vi "Layout Badges.vi"(8 "error in (no error)":errorcluster, 11 "Node in":refnum<class "FSM.Node.lvclass">) -> (0 "error out":errorcluster, 3 "Node out":refnum<class "FSM.Node.lvclass">)   [LabVIEW 2015, in "FSM.Node.lvclass"]
uses:
  FSM.Node.lvclass
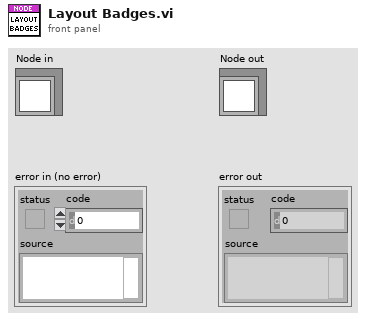
[diagram p1: front panel]
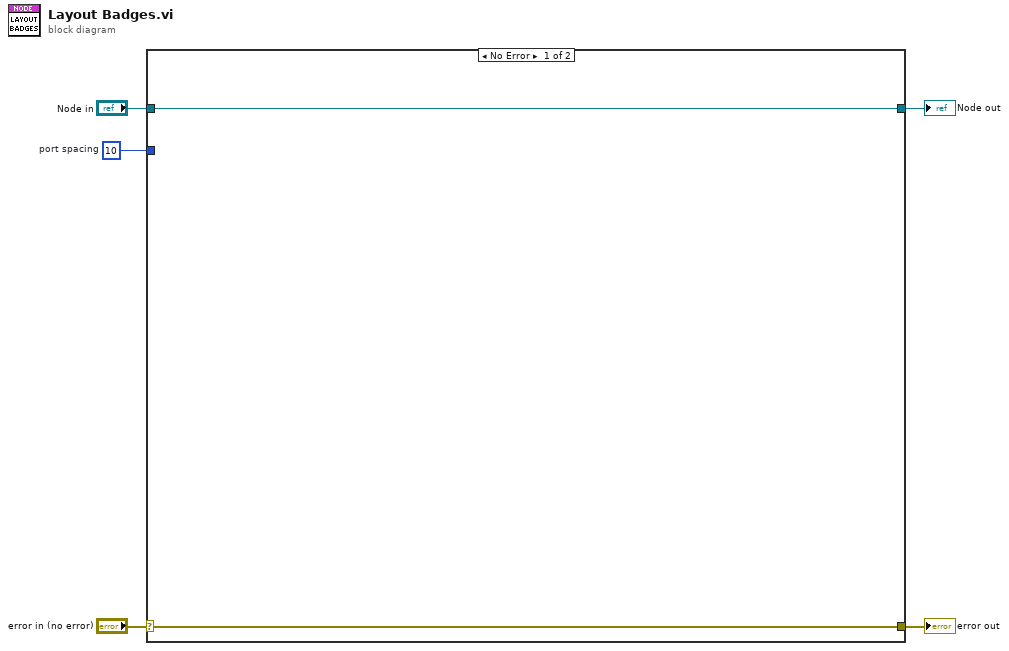
[diagram p0: block diagram]
diagram:
  w1 = 10  # port spacing
  n1 = case shown="No Error" "error in (no error)" {
    selector: "error in (no error)" -> [w7 w9]
    tunnel: [w7 w9] -> w4
    tunnel: [w6 w8] -> w2
    tunnel: "Node in" -> [w6 w8]
    tunnel: w1 -> [_ _]
    frame No Error {
    }
    frame Error {
    }
  }
  "error out" <- w4
  "Node out" <- w2
